vi "SMU Enable.vi"(8 "error in (no error)":errorcluster, 9 "output enabled":bool=TRUE, 10 "Pin":string, 11 "Semiconductor Module Context":T1) -> (0 "error out":errorcluster, 3 "Semiconductor Module Context Out":T1)   [LabVIEW 2013]
uses:
  <vilib>/NI_TestStand_SemiconductorModule/NI_TestStand_Semiconductor_Module.lvlibp/PinMap/General/SemiconductorModuleContext.ctl
  <vilib>/NI_TestStand_SemiconductorModule/NI_TestStand_Semiconductor_Module.lvlibp/PinMap/DC Power/PinToNIDCPowerSession.vi
  <vilib>/NI_TestStand_SemiconductorModule/NI_TestStand_Semiconductor_Module.lvlibp
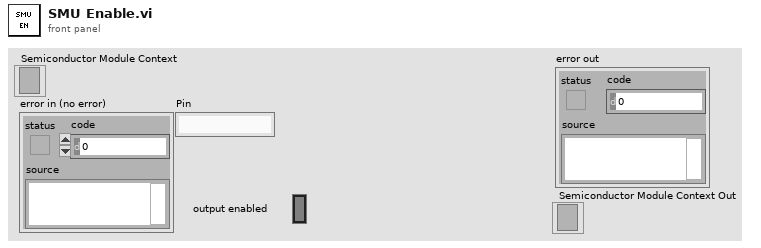
[diagram p1: front panel]
types:
  T1 = typedef "NI_TestStand_Semiconductor_Module.lvlibp/SemiconductorModuleContext.ctl" = refnum<k7>
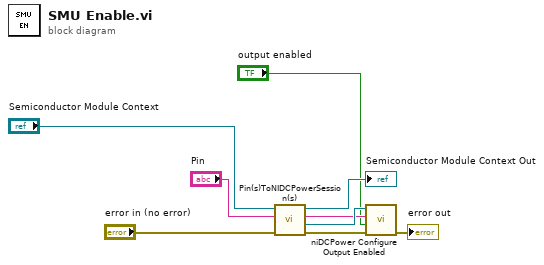
[diagram p0: block diagram]
diagram:
  n1 = call-poly <vilib>:"Pin(s)ToNIDCPowerSession(s).vi"("error in (no error)"="error in (no error)", "Pin"="Pin", "Semiconductor Module Context"="Semiconductor Module Context") -> ("error out"=w2:errorcluster, "Instrument Session"=w5:refnum<k15>, "Channel List"=w4:string, "Semiconductor Module Context Out"=→"Semiconductor Module Context Out":T1)  [unwired: 4 in, 1 out]
  n2 = call <instrlib>:"niDCPower Configure Output Enabled.vi"("error in (no error)"=w2, "output enabled"="output enabled", "channel name"=w4, "instrument handle"=w5) -> ("error out"=→"error out":errorcluster)  [unwired: 6 in, 1 out]
